vi "ROV Test.vi"() -> ()   [LabVIEW 2012]
doc: "This VI serves as a systemwide test case for the Main MATE GUI. When executed with the Main MATE GUI operational and configured, the generated commands from the Main MATE GUI will be observable through the graphics of the rendered steering frame within the front panel.\nRuffin"
uses:
  ROV/Teleop command.ctl
  <vilib>/Platform/TimedLoop/XDataNode/timing_clust.ctl
  <vilib>/Platform/TimedLoop/XDataNode/nitl_modes.ctl
  <vilib>/Platform/TimedLoop/XDataNode/wakeup.ctl
  Support/Robot globals (robot acquires video).vi
  <vilib>/Platform/TimedLoop/XDataNode/XDataNode.xnode
  <vilib>/Platform/TimedLoop/XDataNode/XDNodeRunTimeDep.lvlib
  ROV/ROV Host.lvclass
  <vilib>/robotics/Utilities/NI_Robotics Utilities.lvlib
panel:
  out "Teleop command timed out":bool
  in  "Telemetry":T1(tab)
  out "Teleop command":T2
  out "Comunication Error":errorcluster
  out "Joypad Error":errorcluster
  out "error out":errorcluster
  in  "Error in":errorcluster
  out "Top View":picture
  out "Side View":picture
  in  "Robot Mode:":T3(ring)
  out "Error":bool
  in  "Stop":bool
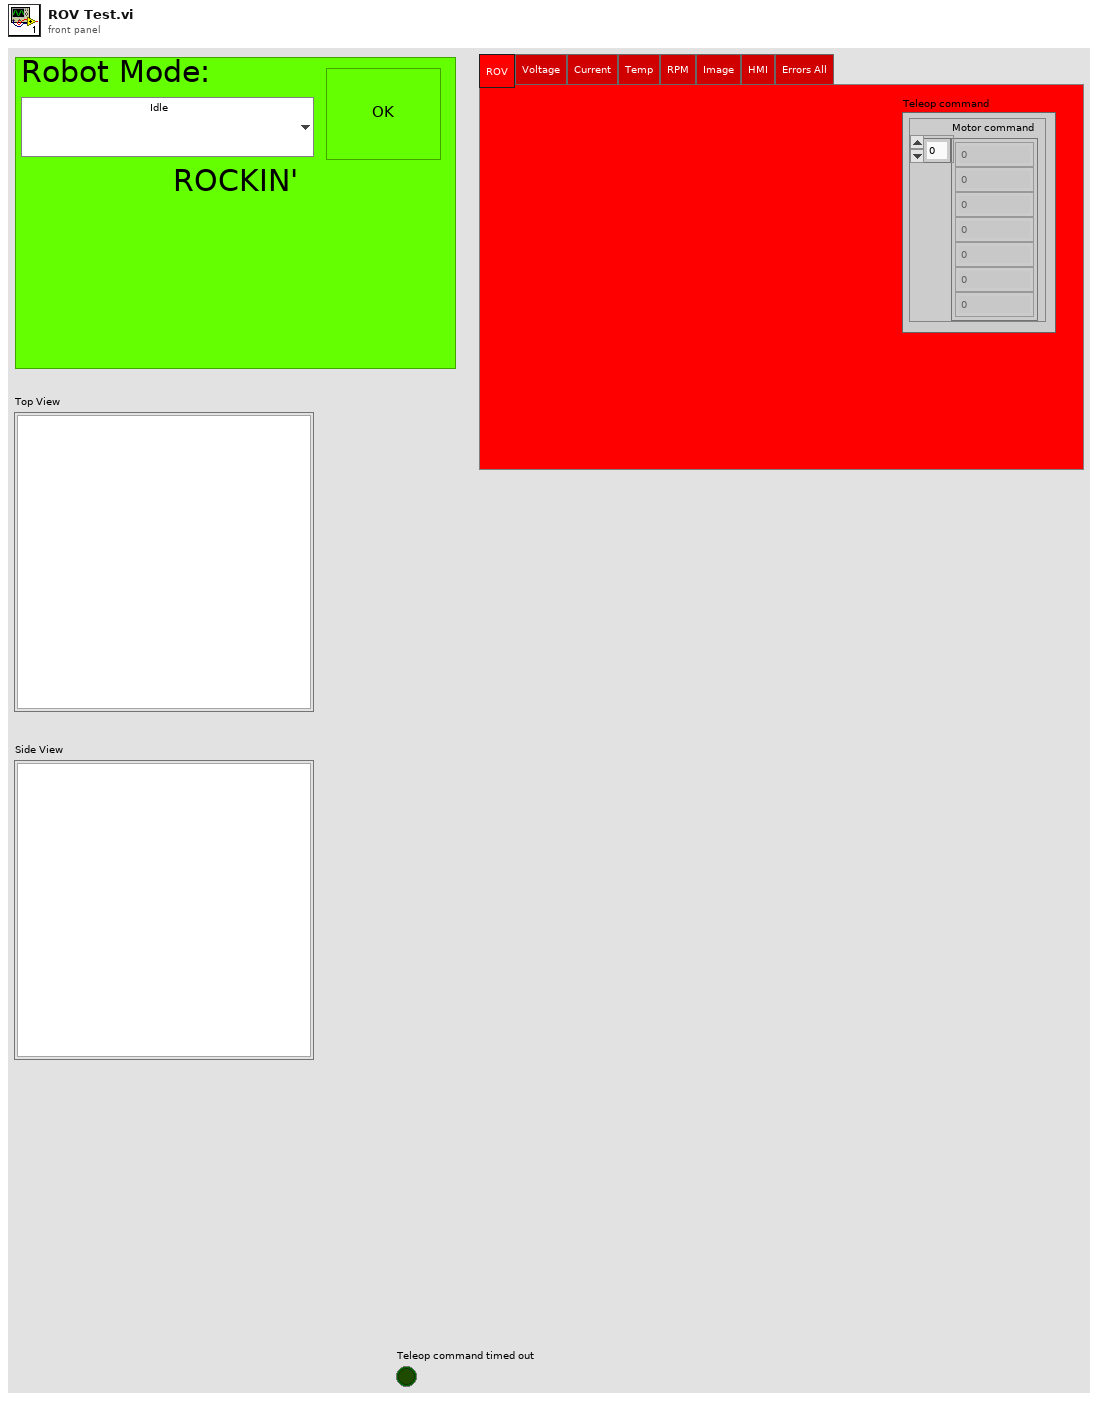
[diagram p1: front panel]
types:
  T1 = enum32{"ROV", "Voltage", "Current", "Temp", "RPM", "Image", "HMI", "Errors All"}
  T2 = typedef "ROV Host.lvclass/Teleop command.ctl" = cluster{"Motor command":dbl[]}
  T3 = enum16{"Idle", "Calibrate", "Teleoperation", "Abort"}
  T4 = typedef "XDNodeRunTimeDep.lvlib/timing_clust.ctl" = cluster{"Expected End [f-1]":u64, "Actual End [f-1]":u64, "Finished Late? [f-1]":bool, "Expected End [i-1]":u64, "Actual End [i-1]":u64, "Finished Late? [i-1]":bool, "Expected Start [i]":u64, "Actual Start [i]":u64, "Expected Start [f]":u64, "Actual Start [f]":u64, "Source Name":string, "Structure Name":string, "Period":i64, "Deadline":i64, "Offset":i64, "Start":i64, "Priority":i32, "Timeout":i32, "Mode":T5, "Wakeup Reason":T6, "Error":errorcluster, "Source Type":string, "Secondary Source Type":string, "Global End Time":u64, "Global Start Time":u64, "Frame Duration":u64, "Iteration Duration":u64, "Assigned CPU":i32, "I/O Scan Engine Mode":u32}
  T5 = typedef "XDNodeRunTimeDep.lvlib/nitl_modes.ctl" = enum32{"No Change", "Process missed periods, maintain original phase", "Discard missed periods, maintain original phase", "Process missed periods, ignore original phase", "Discard missed periods, ignore original phase"}
  T6 = typedef "XDNodeRunTimeDep.lvlib/wakeup.ctl" = enum32{"Normal", "Aborted", "Asynchronous wakeup", "Timing source error", "Timed loop error", "Timeout"}
  T7 = typedef "LVBoundsTypeDef.ctl" = cluster{"Width":u32, "Height":u32}
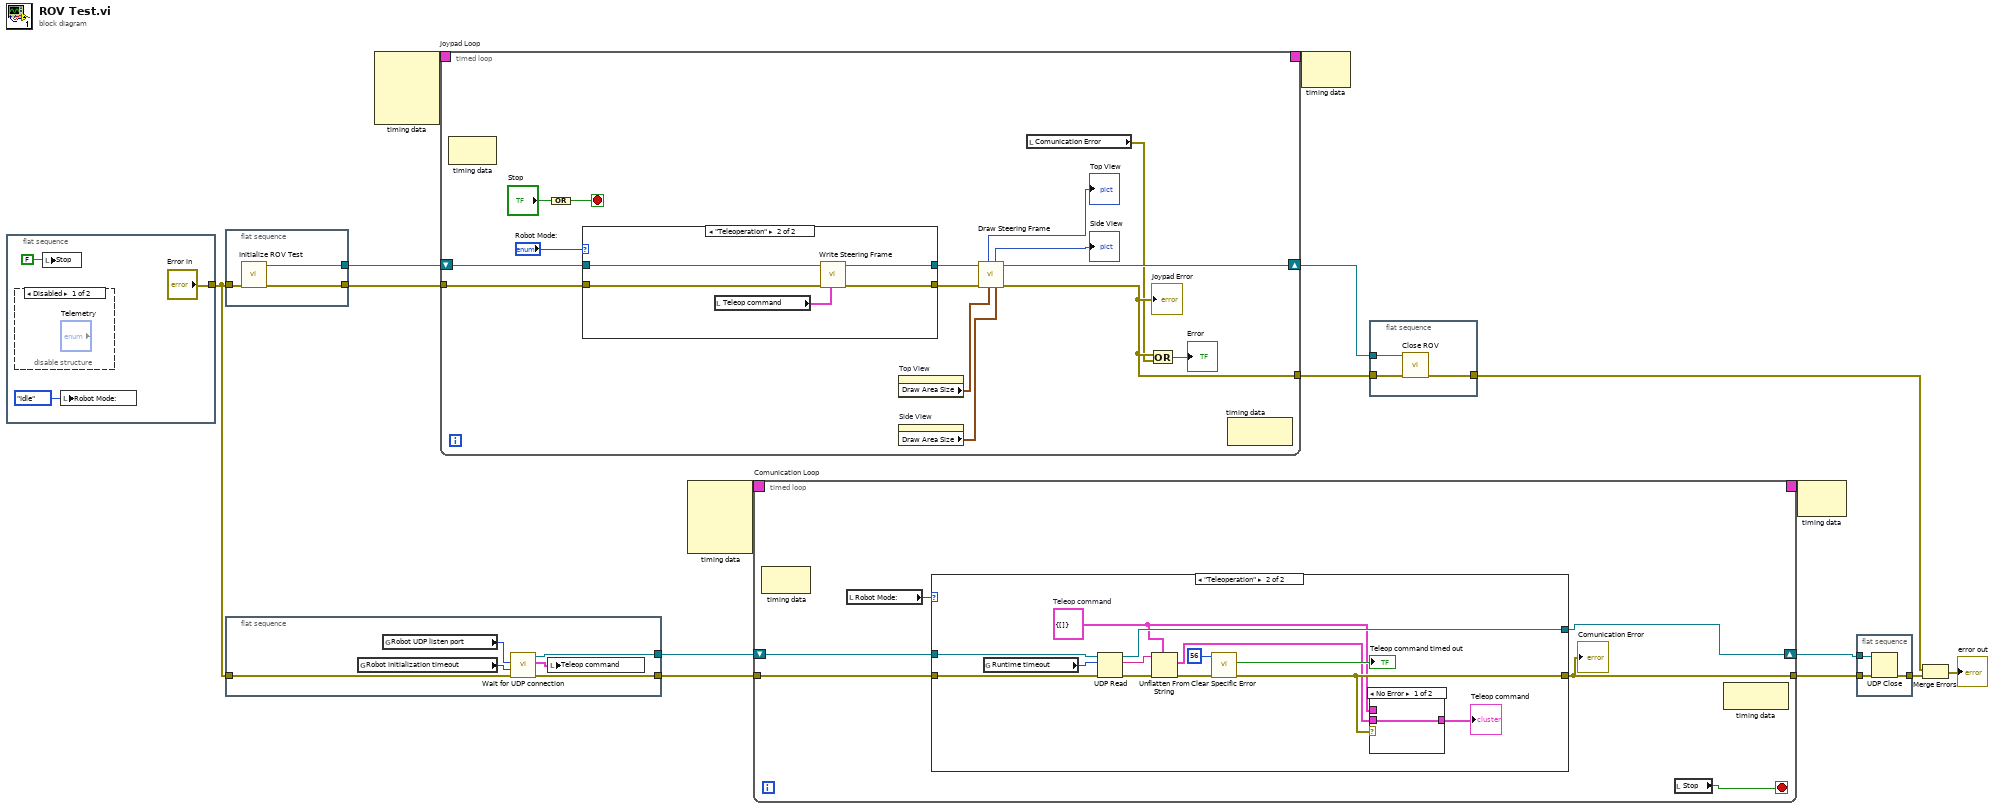
[diagram p0: block diagram]
diagram:
  n1 = flat-sequence {
    tunnel: ["Error in"] -> w5
    frame #0 {
      n2 = disable-structure shown="Disabled" {
        frame Disabled {
        }
        frame Enabled {
        }
      }
      n3 = local write "Stop"(FALSE ("Stop")) -> ()
      n4 = local write "Robot Mode:"(T3."Idle" ("Robot Mode:")) -> ()
    }
  }
  n5 = flat-sequence {
    tunnel: w5 -> [w22]
    tunnel: [w21] -> w2
    tunnel: [w20] -> w1
    frame #0 {
      n6 = call "Initialize ROV Test.vi"("error in (no error)"=w22) -> ("error out"=w21:errorcluster, "ROV Host.lvclass"=w20:refnum<class "ROV Host.lvclass">)  [unwired: 9 in]
    }
  }
  n7 = flat-sequence {
    tunnel: [w28] -> w4
    tunnel: [w27] -> w3
    tunnel: w5 -> [w23]
    frame #0 {
      n8 = global read "Robot globals (robot acquires video).vi" "Robot initialization timeout"() -> (w25:i32)
      n9 = global read "Robot globals (robot acquires video).vi" "Robot UDP listen port"() -> (w26:u16)
      n10 = call "Wait for UDP connection.vi"("error in (no error)"=w23, "Timeout (-1 never timeout)"=w25, "port (60200)"=w26) -> ("error out"=w28:errorcluster, "Initial teleop command"=w24:T2, "UDP Network Connection out"=w27:refnum<k16>)  [unwired: 6 in]
      n11 = local write "Teleop command"(w24) -> ()
    }
  }
  n12 = node-c288() -> (w16:T4)  [unwired: 4 in]
  n13 = timed-loop "Joypad Loop" {
    timing: w16 -> [_]
    timing-out: [_] -> w15
    shift-right: [w34] -> w12
    shift-left: w1 -> [w36]
    tunnel: w2 -> [w41]
    tunnel: [w31] -> w7
    stop <- w43 stop-if-true
    n14 = node-c288() -> ()  [unwired: 1 in, 1 out]
    n15 = Compound Arithmetic op=OR("Stop") -> (w43:bool)
    n16 = case shown="\"Teleoperation\"" "Robot Mode:" {
      tunnel: w41 -> [w45 w49]
      tunnel: [w45 w46] -> w40
      tunnel: w36 -> [w44 w50]
      tunnel: [w44 w47] -> w35
      frame "Idle", Default {
      }
      frame "Teleoperation" {
        n17 = local read "Teleop command"() -> (w48:T2)
        n18 = call "Write Steering Frame.vi"("Teleop command"=w48, "error in (no error)"=w49, "ROV in"=w50) -> ("error out"=w46:errorcluster, "ROV out"=w47:refnum<class "ROV Host.lvclass">)  [unwired: 7 in]
      }
    }
    n19 = property on="Top View" class="Pict"() -> ("Draw Area Size"=w33:T7)  [unwired: 2 in, 2 out]
    n20 = property on="Side View" class="Pict"() -> ("Draw Area Size"=w32:T7)  [unwired: 2 in, 2 out]
    n21 = call "Draw Steering Frame.vi"("Side View Draw Area Size 2"=w32, "Top View Draw Area Size"=w33, "error in (no error)"=w40, "ROV in"=w35) -> ("error out"=w31:errorcluster, "ROV out"=w34:refnum<class "ROV Host.lvclass">, "Side View"=→"Side View":picture, "Top View"=→"Top View":picture)  [unwired: 4 in]
    "Joypad Error" <- w31
    n22 = local read "Comunication Error"() -> (w30:errorcluster)
    n23 = Compound Arithmetic op=OR(w31, w30) -> (→"Error":bool)
    n24 = node-c288() -> ()  [unwired: 1 in, 1 out]
  }
  n25 = node-c288() -> (w14:T4)  [unwired: 4 in]
  n26 = timed-loop "Comunication Loop" {
    timing: w14 -> [_]
    timing-out: [_] -> w13
    shift-right: [w54] -> w10
    shift-left: w3 -> [w53]
    tunnel: w4 -> [w56]
    tunnel: [w55] -> w11
    stop <- w57 stop-if-true
    n27 = node-c288() -> ()  [unwired: 1 in, 1 out]
    n28 = local read "Robot Mode:"() -> (w58:T3)
    n29 = case shown="\"Teleoperation\"" w58 {
      tunnel: w56 -> [w60 w67]
      tunnel: [w60 w64] -> w55
      tunnel: w53 -> [w59 w66]
      tunnel: [w59 w65] -> w54
      frame "Idle", Default {
      }
      frame "Teleoperation" {
        w62 = T2 {"Motor command"=[]}  # Teleop command
        n30 = global read "Robot globals (robot acquires video).vi" "Runtime timeout"() -> (w68:i32)
        n31 = UDP Read(connection ID=w66, max size (548)=w68, 8:w67) -> (data out=w69:string, error out=w70:errorcluster, 3:w65:refnum<k16>)  [unwired: 1 in, 2 out]
        n32 = Unflatten From String(type=w62, binary string=w69, error in (no error)=w70) -> (value=w61:T2, error out=w72:errorcluster)  [unwired: 2 in, 1 out]
        n33 = call <vilib>:"Clear Specific Error.vi"("error in (no error)"=w72, "code"=56) -> ("error out"=w64:errorcluster, "cleared?"=→"Teleop command timed out":bool)  [unwired: 7 in, 1 out]
        n34 = case shown="No Error" w64 {
          tunnel: [w74 w75] -> w63
          tunnel: w61 -> [w74 _]
          tunnel: w62 -> [_ w75]
          frame No Error {
          }
          frame Error {
          }
        }
        "Teleop command" <- w63
      }
    }
    "Comunication Error" <- w55
    n35 = local read "Stop"() -> (w57:bool)
    n36 = node-c288() -> ()  [unwired: 1 in, 1 out]
  }
  n37 = node-c288(w15) -> ()  [unwired: 1 out]
  n38 = flat-sequence {
    tunnel: w12 -> [w80]
    tunnel: w7 -> [w79]
    tunnel: [w78] -> w8
    frame #0 {
      n39 = call "Close ROV.vi"("error in (no error)"=w79, "ROV in"=w80) -> ("error out"=w78:errorcluster)  [unwired: 9 in]
    }
  }
  n40 = node-c288(w13) -> ()  [unwired: 1 out]
  n41 = flat-sequence {
    tunnel: w11 -> [w83]
    tunnel: [w82] -> w9
    tunnel: w10 -> [w81]
    frame #0 {
      n42 = UDP Close(connection ID=w81, 8:w83) -> (error out=w82:errorcluster)  [unwired: 1 out]
    }
  }
  n43 = Merge Errors(w8, w9) -> (→"error out":errorcluster)
